vi "Prj1_Main.vi"() -> ()   [LabVIEW 2020]
doc: "Use this template to build a producer/consumer design pattern with events to produce queue items. Use this design pattern instead of the User Interface Event Handler pattern for user interfaces when you want to execute code asynchronously in response to an event without slowing the user interface responsiveness."
uses:
  <vilib>/Instr/_visa.llb/VISA Configure Serial Port (Instr).vi
panel:
  out "previous error":dbl
  out "previous itegrtion error":dbl
  in  "init Integral? (F)":bool
  in  "Use PID":bool
  out "output":dbl format="%.2f"
  in  "PID gains":T1={"proportional gain (Kc)"=1.0, "integral time (Ti, min)"=0.01, "derivative time (Td, min)"=0.0} {"derivative time (Td, min)" format="%.3f"; "integral time (Ti, min)" format="%.6f"; "proportional gain (Kc)" format="%.3f"}
  out "Motor Feedback Speed (RPM)":dbl
  out "Motor Feedback Speed":dbl(knob) scale=0.0..20.0
  in  "Set Speed":dbl(slide) scale=0.0..15.0
  out "Data Read from Serial Port (Motor Feedback Speed)":string
  in  "Baud rate (9600)":u32=9600
  in  "Serial Port name":refnum<visa-resource-name>
  in  "Close":bool
  in  "Open":bool
  out "Connected":bool
  in  "stop":bool
  # "User Interface / Control Panel"
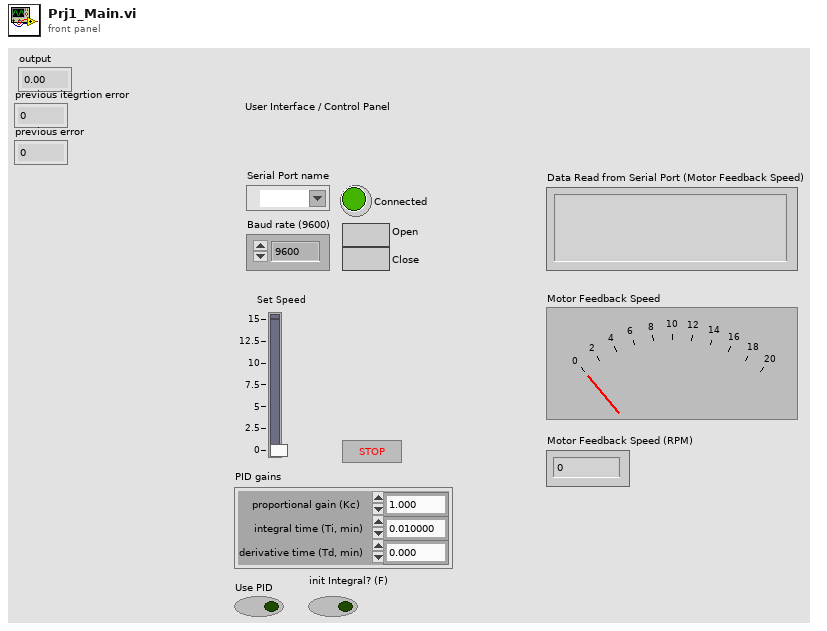
[diagram p1: front panel]
types:
  T1 = cluster{"proportional gain (Kc)":dbl, "integral time (Ti, min)":dbl, "derivative time (Td, min)":dbl}
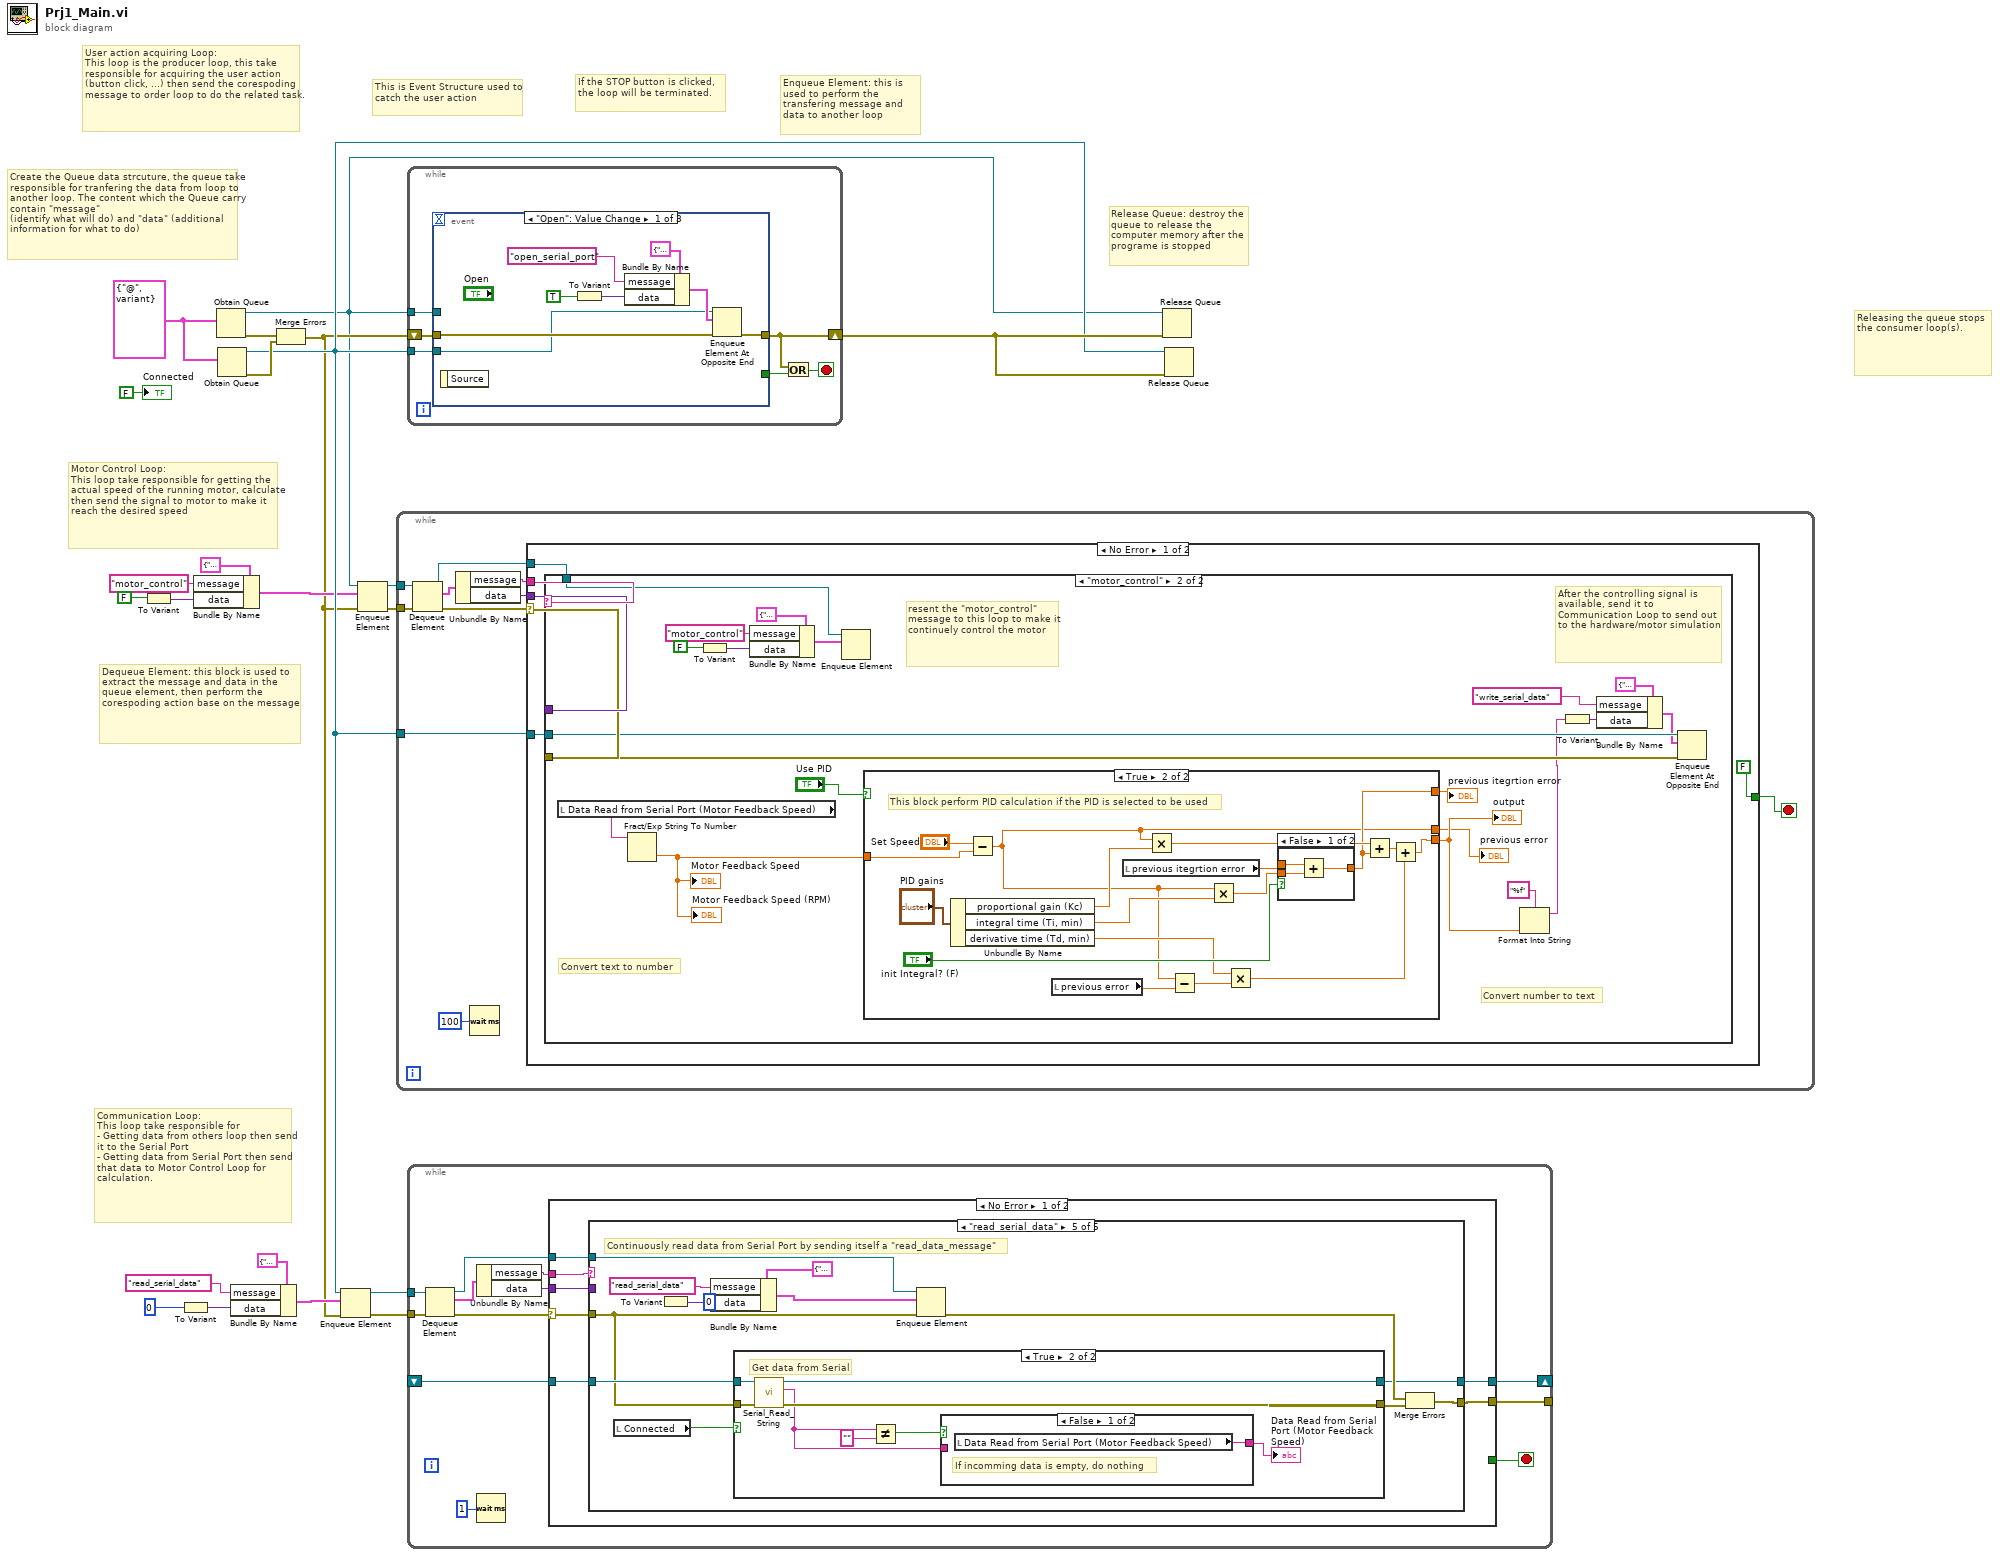
[diagram p0: block diagram]
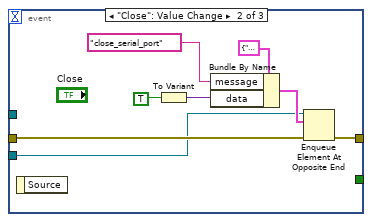
[diagram p2: hidden frame]
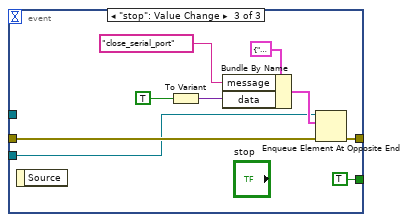
[diagram p3: hidden frame]
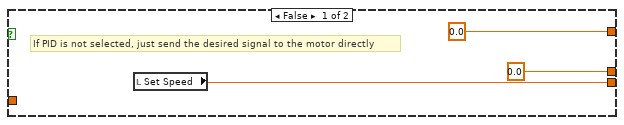
[diagram p5: hidden frame]
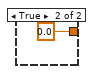
[diagram p6: hidden frame]
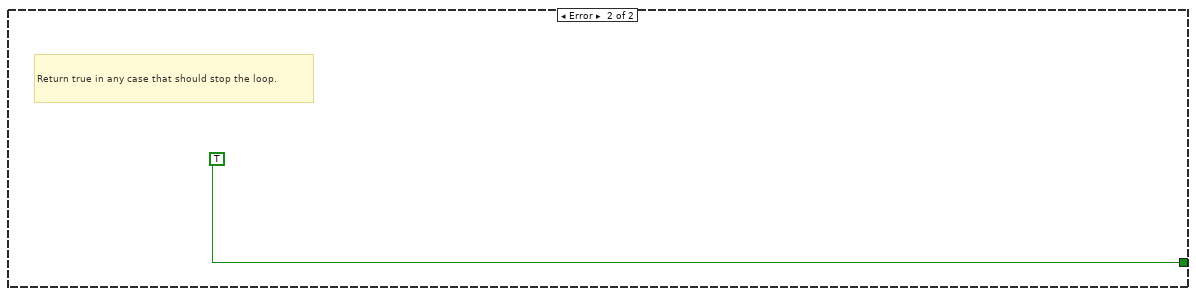
[diagram p7: hidden frame]
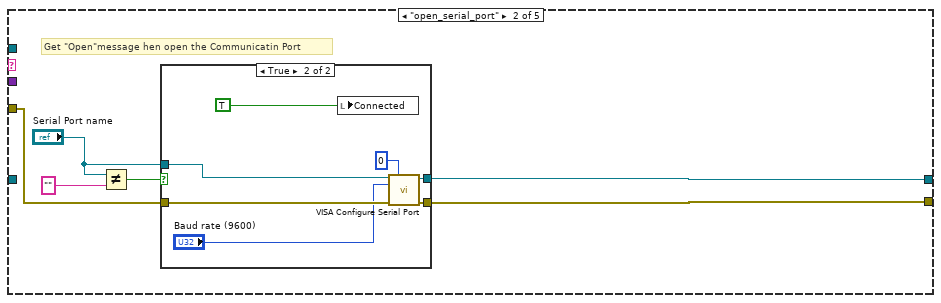
[diagram p9: hidden frame]
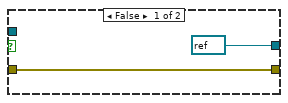
[diagram p10: hidden frame]
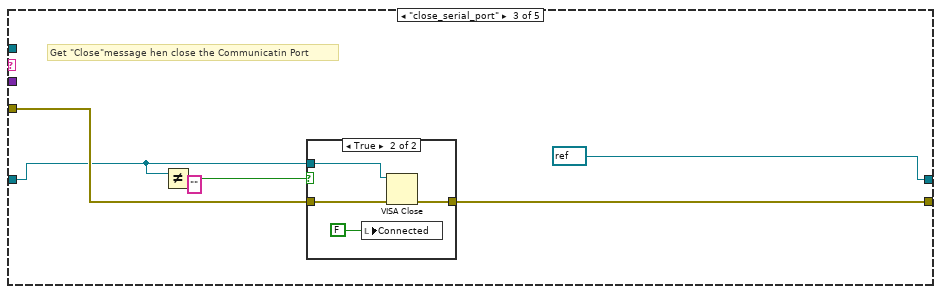
[diagram p11: hidden frame]
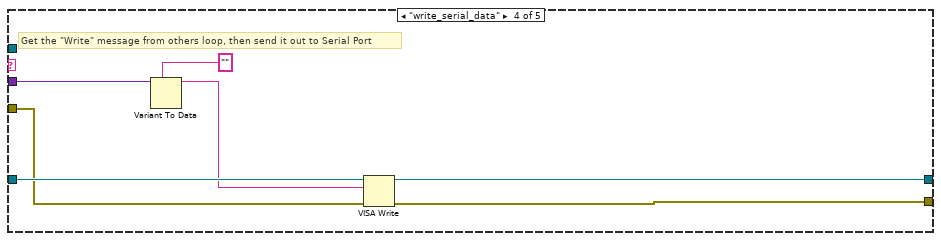
[diagram p13: hidden frame]
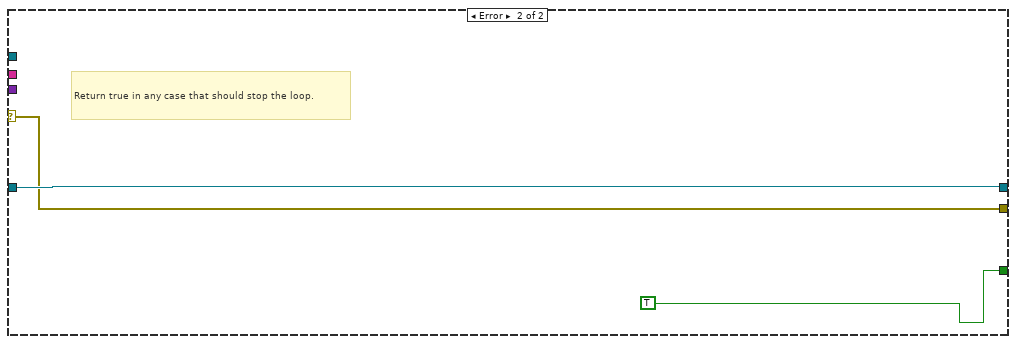
[diagram p16: hidden frame]
diagram:
  w21 = cluster{"message":string, "data":variant} {"message"="@", "data"=variant}
  # "Communication Loop:\nThis loop take responsible for \n- Getting data from others loop then send it to the Serial Port\n- Getting data from Serial Port then send that data to Motor Control Loop for calculation."
  # "Dequeue Element: this block is used to extract the message and data in the queue element, then perform the corespoding action base on the message"
  # "Motor Control Loop:\nThis loop take responsible for getting the actual speed of the running motor, calculate then send the signal to motor to make it reach the desired speed"
  # "Release Queue: destroy the queue to release the computer memory after the programe is stopped"
  # "Enqueue Element: this is used to perform the transfering message and data to another loop"
  # "If the STOP button is clicked, the loop will be terminated."
  # "Create the Queue data strcuture, the queue take responsible for tranfering the data from loop to another loop. The content which the Queue carry contain \"message\" \n(identify what will do) and \"data\" (additional information for what to do)"
  # "This is Event Structure used to catch the user action"
  # "User action acquiring Loop:\nThis loop is the producer loop, this take responsible for acquiring the user action (button click, ...) then send the corespoding message to order loop to do the related task."
  # "Releasing the queue stops the consumer loop(s)."
  n1 = To Variant(anything=FALSE ("Write Data")) -> (Variant=w9:variant)
  n2 = To Variant(anything=0) -> (Variant=w14:variant)
  n3 = Bundle By Name(cluster=cluster{"message":string, "data":variant} {"message"="@", "data"=variant}, "message"="motor_control", "data"=w9) -> (w8:cluster{"message":string, "data":variant})
  n4 = Obtain Queue(element data type=w21) -> (queue out=w1:refnum<queue>, error out=w20:errorcluster)  [unwired: 4 in, 1 out]
  n5 = Obtain Queue(element data type=w21) -> (queue out=w10:refnum<queue>, error out=w19:errorcluster)  [unwired: 4 in, 1 out]
  n6 = Bundle By Name(cluster=cluster{"message":string, "data":variant} {"message"="@", "data"=variant}, "message"="read_serial_data", "data"=w14) -> (w17:cluster{"message":string, "data":variant})
  n7 = Merge Errors(w20, w19) -> (w3:errorcluster)
  n8 = Enqueue Element(queue=w10, element=w17, error in (no error)=w3) -> (queue out=w11:refnum<queue>, error out=w12:errorcluster)  [unwired: 1 in, 1 out]
  n9 = Enqueue Element(queue=w1, element=w8, error in (no error)=w3) -> (queue out=w2:refnum<queue>, error out=w4:errorcluster)  [unwired: 1 in, 1 out]
  n10 = while {
    tunnel: w2 -> [w32]
    tunnel: w4 -> [w28]
    tunnel: w10 -> [w25]
    stop <- w30 stop-if-true
    n11 = Dequeue Element(queue=w32, error in (no error)=w28) -> (queue out=w24:refnum<queue>, element=w29:cluster{"message":string, "data":variant}, error out=w31:errorcluster)  [unwired: 1 in, 1 out]
    n12 = Unbundle By Name(w29) -> ("message"=w27:string, "data"=w26:variant)
    n13 = Wait (ms)(milliseconds to wait=u32 100) -> ()  [unwired: 1 out]
    n14 = case shown="No Error" w31 {
      selector: w31 -> [w36 _]
      tunnel: [FALSE TRUE] -> w30
      tunnel: w27 -> [w38 _]
      tunnel: w26 -> [w37 _]
      tunnel: w25 -> [w35 _]
      tunnel: w24 -> [w33 _]
      frame No Error {
        n15 = case shown="\"motor_control\"" w38 {
          tunnel: w37 -> [_ _]
          tunnel: w36 -> [_ w57]
          tunnel: w35 -> [_ w58]
          tunnel: w33 -> [_ w43]
          frame "False", Default {
          }
          frame "motor_control" {
            # "Convert number to text"
            # "Convert text to number"
            # "After the controlling signal is available, send it to Communication Loop to send out to the hardware/motor simulation"
            # "resent the \"motor_control\" message to this loop to make it continuely control the motor"
            n16 = local read "Data Read from Serial Port (Motor Feedback Speed)"() -> (w50:string)
            n17 = Fract/Exp String To Number(string=w50) -> (number=w48:dbl)  [unwired: 3 in, 1 out]
            "Motor Feedback Speed" <- w48
            "Motor Feedback Speed (RPM)" <- w48
            n18 = To Variant(anything=FALSE ("Write Data")) -> (Variant=w55:variant)
            n19 = Bundle By Name(cluster=cluster{"message":string, "data":variant} {"message"="@", "data"=variant}, "message"="motor_control", "data"=w55) -> (w54:cluster{"message":string, "data":variant})
            n20 = Enqueue Element(queue=w43, element=w54) -> ()  [unwired: 2 in, 3 out]
            n21 = case shown="True" "Use PID" {
              tunnel: w48 -> [_ w77]
              tunnel: [w61 w66] -> w47
              tunnel: [0.0 w71] -> w45
              tunnel: [0.0 w62] -> w44
              frame False {
                # "If PID is not selected, just send the desired signal to the motor directly"
                n22 = local read "Set Speed"() -> (w61:dbl)
              }
              frame True {
                # "This block perform PID calculation if the PID is selected to be used"
                n23 = Unbundle By Name("PID gains") -> ("proportional gain (Kc)"=w75:dbl, "integral time (Ti, min)"=w64:dbl, "derivative time (Td, min)"=w68:dbl)
                n24 = Subtract(x="Set Speed", y=w77) -> (x-y=w62:dbl)
                n25 = local read "previous error"() -> (w63:dbl)
                n26 = local read "previous itegrtion error"() -> (w74:dbl)
                n27 = Multiply(x=w62, y=w75) -> (x*y=w73:dbl)
                n28 = Subtract(x=w62, y=w63) -> (x-y=w69:dbl)
                n29 = Multiply(x=w62, y=w64) -> (x*y=w70:dbl)
                n30 = Multiply(x=w68, y=w69) -> (x*y=w65:dbl)
                n31 = case shown="False" "init Integral? (F)" {
                  tunnel: w74 -> [w81 _]
                  tunnel: w70 -> [w80 _]
                  tunnel: [w79 0.0] -> w71
                  frame False {
                    n32 = Add(x=w81, y=w80) -> (x+y=w79:dbl)
                  }
                  frame True {
                  }
                }
                n33 = Add(x=w73, y=w71) -> (x+y=w67:dbl)
                n34 = Add(x=w67, y=w65) -> (x+y=w66:dbl)
              }
            }
            "output" <- w47
            "previous itegrtion error" <- w45
            "previous error" <- w44
            n35 = Format Into String(format string="%f", w47) -> (resulting string=w49:string)  [unwired: 2 in, 1 out]
            n36 = To Variant(anything=w49) -> (Variant=w39:variant)
            n37 = Bundle By Name(cluster=cluster{"message":string, "data":variant} {"message"="@", "data"=variant}, "message"="write_serial_data", "data"=w39) -> (w42:cluster{"message":string, "data":variant})
            n38 = Enqueue Element At Opposite End(queue=w58, element=w42, error in (no error)=w57) -> ()  [unwired: 1 in, 3 out]
          }
        }
      }
      frame Error {
        # "Return true in any case that should stop the loop."
      }
    }
  }
  n39 = while {
    shift-right: [w85] -> w18
    shift-left: w3 -> [w88]
    tunnel: w1 -> [w89]
    tunnel: w10 -> [w84]
    stop <- w86 stop-if-true
    n40 = event shown="[0] \"Open\": Value Change" {
      selector: _ -> [_ _ _]
      dyn-events: _ -> [_ _ _]
      timeout: _ -> [_ _ _]
      tunnel: w89 -> [_ _ _]
      tunnel: w88 -> [w93 w101 w110]
      tunnel: [w92 w100 w109] -> w85
      tunnel: [_ _ TRUE ("stop")] -> w87
      tunnel: w84 -> [w91 w99 w108]
      event "Open": Value Change {
        n41 = event-data() -> ()  [unwired: 1 in, 1 out]
        n42 = To Variant(anything=TRUE ("Open")) -> (Variant=w94:variant)
        n43 = Bundle By Name(cluster=cluster{"message":string, "data":variant} {"message"="@", "data"=variant}, "message"="open_serial_port", "data"=w94) -> (w97:cluster{"message":string, "data":variant})
        n44 = Enqueue Element At Opposite End(queue=w91, element=w97, error in (no error)=w93) -> (error out=w92:errorcluster)  [unwired: 1 in, 2 out]
      }
      event "Close": Value Change {
        n45 = event-data() -> ()  [unwired: 1 in, 1 out]
        n46 = To Variant(anything=TRUE ("Close")) -> (Variant=w102:variant)
        n47 = Bundle By Name(cluster=cluster{"message":string, "data":variant} {"message"="@", "data"=variant}, "message"="close_serial_port", "data"=w102) -> (w105:cluster{"message":string, "data":variant})
        n48 = Enqueue Element At Opposite End(queue=w99, element=w105, error in (no error)=w101) -> (error out=w100:errorcluster)  [unwired: 1 in, 2 out]
      }
      event "stop": Value Change {
        n49 = event-data() -> ()  [unwired: 1 in, 1 out]
        n50 = To Variant(anything=TRUE ("stop")) -> (Variant=w111:variant)
        n51 = Bundle By Name(cluster=cluster{"message":string, "data":variant} {"message"="@", "data"=variant}, "message"="close_serial_port", "data"=w111) -> (w114:cluster{"message":string, "data":variant})
        n52 = Enqueue Element At Opposite End(queue=w108, element=w114, error in (no error)=w110) -> (error out=w109:errorcluster)  [unwired: 1 in, 2 out]
      }
    }
    n53 = Or(x=w85, y=w87) -> (x .or. y?=w86:bool)
  }
  n54 = while {
    tunnel: w11 -> [w126]
    tunnel: w12 -> [w122]
    shift-right: [w119] -> _
    shift-left: _ -> [w118]
    tunnel: [w117] -> _
    stop <- w124 stop-if-true
    n55 = Dequeue Element(queue=w126, error in (no error)=w122) -> (queue out=w116:refnum<queue>, element=w123:cluster{"message":string, "data":variant}, error out=w125:errorcluster)  [unwired: 1 in, 1 out]
    n56 = Unbundle By Name(w123) -> ("message"=w121:string, "data"=w120:variant)
    n57 = Wait (ms)(milliseconds to wait=u32 1) -> ()  [unwired: 1 out]
    n58 = case shown="No Error" w125 {
      selector: w125 -> [w131 w194]
      tunnel: [_ TRUE] -> w124
      tunnel: w121 -> [w133 _]
      tunnel: w120 -> [w132 _]
      tunnel: [w130 w195] -> w119
      tunnel: w118 -> [w129 w195]
      tunnel: [w128 w194] -> w117
      tunnel: w116 -> [w127 _]
      frame No Error {
        n59 = case shown="\"read_serial_data\"" w133 {
          tunnel: w132 -> [_ _ _ w163 _]
          tunnel: w131 -> [w134 w141 w156 w166 w174]
          tunnel: [w135 w137 refnum<visa-resource-name> refnum ("VISA resource name out") w165 w170] -> w130
          tunnel: w129 -> [w135 _ w151 w168 w175]
          tunnel: [w134 w136 w153 w164 w171] -> w128
          tunnel: w127 -> [_ _ _ _ w177]
          frame "False", Default {
            # "If there are no message come, doing nothing"
          }
          frame "open_serial_port" {
            # "Get \"Open\"message hen open the Communicatin Port"
            n60 = Not Equal?(x="Serial Port name", y="") -> (x != y?=w139:bool)
            n61 = case shown="True" w139 {
              tunnel: w141 -> [w142 w149]
              tunnel: "Serial Port name" -> [_ w146]
              tunnel: [refnum<visa-resource-name> refnum ("VISA resource name") w147] -> w137
              tunnel: [w142 w148] -> w136
              frame False {
              }
              frame True {
                n62 = local write "Connected"(TRUE ("Boolean")) -> ()
                n63 = call-poly "VISA Configure Serial Port"("VISA resource name"=w146, "timeout (10sec)"=u32 0, "baud rate (9600)"="Baud rate (9600)", "error in (no error)"=w149) -> ("VISA resource name out"=w147:refnum<visa-resource-name>, "error out"=w148:errorcluster)  [unwired: 10 in]
              }
            }
          }
          frame "close_serial_port" {
            # "Get \"Close\"message hen close the Communicatin Port"
            n64 = Not Equal?(x=w151, y="") -> (x != y?=w154:bool)
            n65 = case shown="True" w154 {
              tunnel: w156 -> [w157 w161]
              tunnel: w151 -> [_ w160]
              tunnel: [w157 w158] -> w153
              frame False {
              }
              frame True {
                n66 = local write "Connected"(FALSE ("Boolean")) -> ()
                n67 = VISA Close(VISA resource name=w160, error in (no error)=w161) -> (error out=w158:errorcluster)
              }
            }
          }
          frame "write_serial_data" {
            # "Get the \"Write\" message from others loop, then send it out to Serial Port"
            n68 = Variant To Data(type="", Variant=w163) -> (data=w167:string)  [unwired: 1 in, 1 out]
            n69 = VISA Write(VISA resource name=w168, write buffer=w167, error in (no error)=w166) -> (VISA resource name out=w165:refnum<visa-resource-name>, error out=w164:errorcluster)  [unwired: 1 out]
          }
          frame "read_serial_data" {
            # "Continuously read data from Serial Port by sending itself a \"read_data_message\""
            n70 = local read "Connected"() -> (w169:bool)
            n71 = To Variant(anything=0) -> (Variant=w178:variant)
            n72 = Bundle By Name(cluster=cluster{"message":string, "data":variant} {"message"="@", "data"=variant}, "message"="read_serial_data", "data"=w178) -> (w181:cluster{"message":string, "data":variant})
            n73 = case shown="True" w169 {
              tunnel: w175 -> [w183 w189]
              tunnel: w174 -> [w182 w188]
              tunnel: [w182 w191] -> w172
              tunnel: [w183 w190] -> w170
              frame False {
              }
              frame True {
                # "Get data from Serial"
                n74 = call "Serial_Read_String.vi"("error in (no error)"=w188, "VISA Refnum in"=w189) -> ("error out"=w191:errorcluster, "read buffer"=w186:string, "VISA Refnum out"=w190:refnum<visa-resource-name>)  [unwired: 7 in]
                n75 = Not Equal?(x=w186, y="") -> (x != y?=w185:bool)
                n76 = case shown="False" w185 {
                  tunnel: [w192 w193] -> w184
                  tunnel: w186 -> [_ w193]
                  frame False {
                    # "If incomming data is empty, do nothing"
                    n77 = local read "Data Read from Serial Port (Motor Feedback Speed)"() -> (w192:string)
                  }
                  frame True {
                    # "If incomming data the vailed, get it"
                  }
                }
                "Data Read from Serial Port (Motor Feedback Speed)" <- w184
              }
            }
            n78 = Enqueue Element(queue=w177, element=w181, error in (no error)=w174) -> (error out=w173:errorcluster)  [unwired: 1 in, 2 out]
            n79 = Merge Errors(w173, w172) -> (w171:errorcluster)
          }
        }
      }
      frame Error {
        # "Return true in any case that should stop the loop."
      }
    }
  }
  n80 = Release Queue(queue=w1, error in (no error)=w18) -> ()  [unwired: 1 in, 3 out]
  n81 = Release Queue(queue=w10, error in (no error)=w18) -> ()  [unwired: 1 in, 3 out]
  "Connected" <- FALSE ("Boolean")
